vi "Tube Areas.vi"(10 "NDHX Tube Length (m)":dbl, 11 "NDHX Tube Diameter (m)":dbl) -> (0 "Wall Thickness (m)":dbl, 1 "Am":dbl, 2 "Ai":dbl, 3 "Ao":dbl)   [LabVIEW 2019]
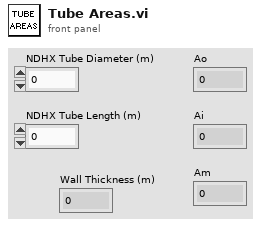
[diagram p1: front panel]
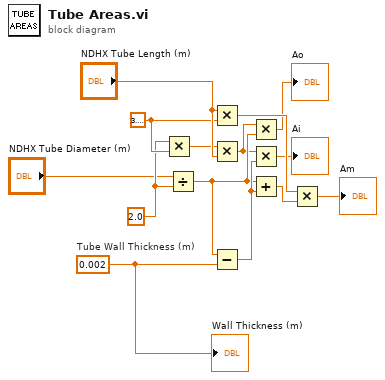
[diagram p0: block diagram]
diagram:
  w8 = 3.141592653589793
  w3 = 2.0 ("y")
  w1 = 0.002  # Tube Wall Thickness (m)
  n1 = Multiply(x=w3, y=w8) -> (x*y=w4:dbl)
  n2 = Divide(x="NDHX Tube Diameter (m)", y=w3) -> (x/y=w11:dbl)
  n3 = Multiply(x="NDHX Tube Length (m)", y=w8) -> (x*y=w10:dbl)
  n4 = Multiply(x=w4, y="NDHX Tube Length (m)") -> (x*y=w5:dbl)
  n5 = Subtract(x=w11, y=w1) -> (x-y=w12:dbl)
  n6 = Multiply(x=w5, y=w11) -> (x*y=→"Ao":dbl)
  n7 = Multiply(x=w5, y=w12) -> (x*y=→"Ai":dbl)
  n8 = Add(x=w11, y=w12) -> (x+y=w13:dbl)
  n9 = Multiply(x=w10, y=w13) -> (x*y=→"Am":dbl)
  "Wall Thickness (m)" <- w1
